vi "AIT 1553 Message Page.vi"(8 "error in (no error)":errorcluster, 11 "Node Ptr":T1 format="%.0x") -> (0 "error out":errorcluster)   [LabVIEW 2011, in "AIT 1553 Custom Device.lvlib"]
uses:
  AIT 1553 Custom Device.lvlib
  <vilib>/NI Veristand/Custom Device API/Custom Device Item Ref.ctl
  Controls and Global/Global.vi
  <vilib>/NI Veristand/Custom Device API/Get Item Property (U32 Array).vi
  <vilib>/NI Veristand/Custom Device API/Get Item Property (Boolean).vi
  <vilib>/NI Veristand/Custom Device API/Get Item Property (U16).vi
  <vilib>/NI Veristand/Custom Device API/Custom Device API.lvlib
panel:
  out "Default Message Buffer Data":u32[](array[numeric])
  out "Messge Buffer ID":u16
  out "RT Sub Address":u16
  out "RT Address":u16
  out "Message Type":string
  in  "Header":cluster{"Section Name":string}={"Section Name"="AIT 1553 Message"}
  in  "Description":string
  out "Name":string
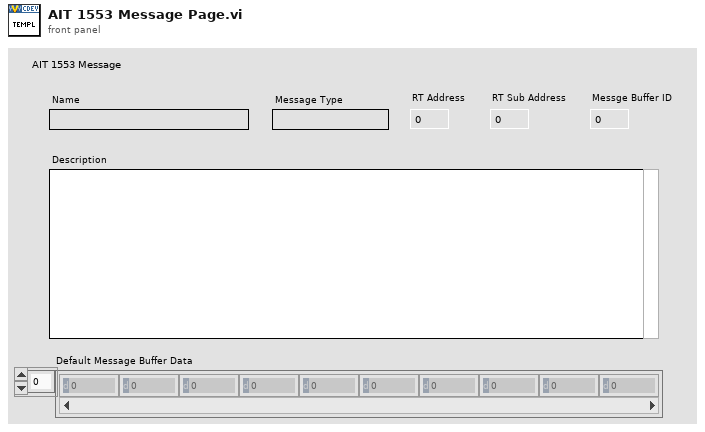
[diagram p1: front panel]
types:
  T1 = typedef "Custom Device API.lvlib/Custom Device Item Ref.ctl" = u64
  T2 = typedef "Custom Device API.lvlib/Custom Device Item Info.ctl" = cluster{"Name":string, "Is Channel":bool, "GUID":string}
  T3 = typedef "Custom Device API.lvlib/Custom Device Commands.ctl" = enum16{"Default", "Item renamed", "Shutdown", "Dynamic button pressed"}
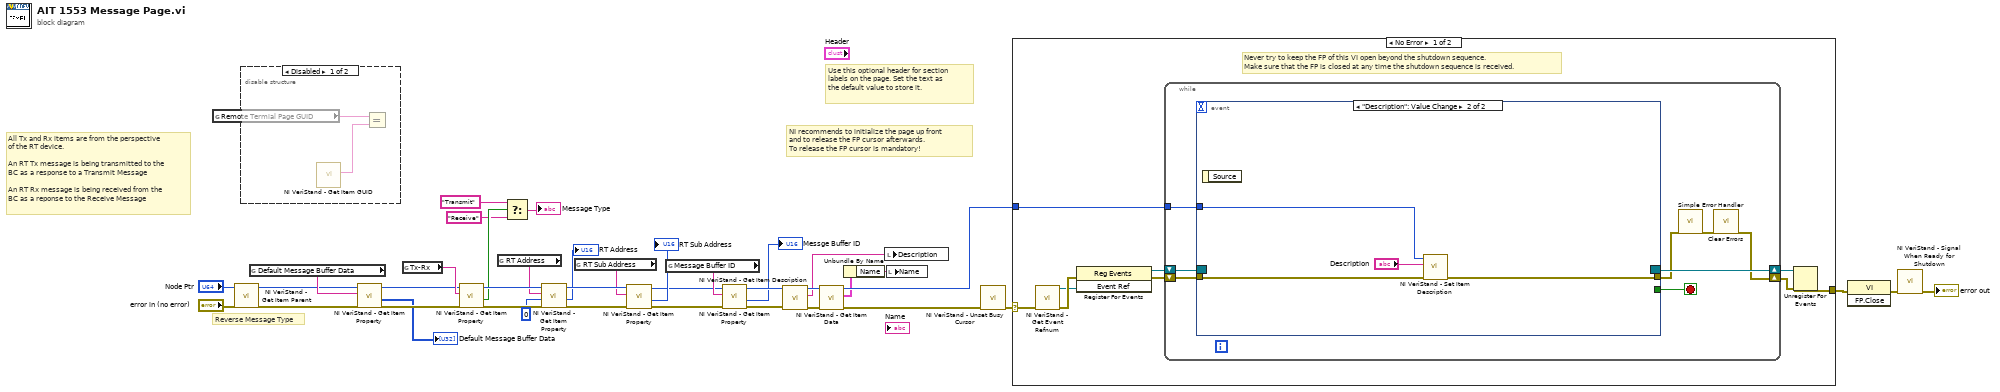
[diagram p0: block diagram]
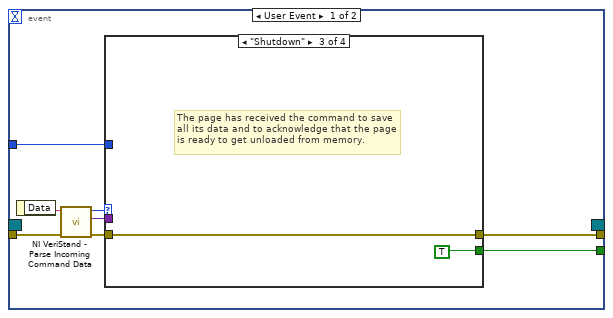
[diagram p3: hidden frame]
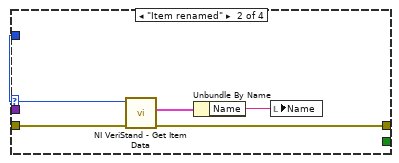
[diagram p5: hidden frame]
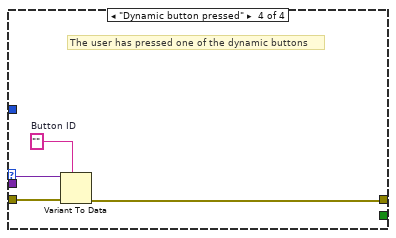
[diagram p6: hidden frame]
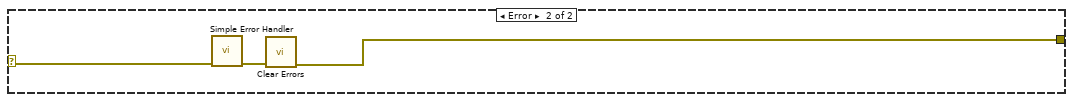
[diagram p7: hidden frame]
diagram:
  # "Reverse Message Type"
  # "All Tx and Rx items are from the perspective \nof the RT device.\n\nAn RT Tx message is being transmitted to the \nBC as a response to a Transmit Message\n\nAn RT Rx message is being received from the \nBC as a reponse to the Receive Message"
  # "Use this optional header for section labels on the page. Set the text as the default value to store it."
  # "NI recommends to initialize the page up front\nand to release the FP cursor afterwards.\nTo release the FP cursor is mandatory!"
  n1 = call <vilib>:"NI VeriStand - Get Item Parent.vi"("error in (no error)"="error in (no error)", "Item Ref in"="Node Ptr") -> ("error out"=w2:errorcluster, "Item Ref out"=w1:T1)  [unwired: 6 in, 2 out]
  n2 = disable-structure shown="Disabled" {
    frame Disabled {
      n3 = global read "Global.vi" "Remote Termial Page GUID"() -> (w40:string)
      n4 = call <vilib>:"NI VeriStand - Get Item GUID.vi"() -> ("GUID"=w41:string)  [unwired: 9 in, 2 out]
      n5 = Equal?(x=w40, y=w41) -> ()  [unwired: 1 out]
    }
    frame Enabled {
    }
  }
  n6 = global read "Global.vi" "Default Message Buffer Data"() -> (w5:string)
  n7 = call-poly <vilib>:"NI VeriStand - Get Item Property.vi"("error in (no error)"=w2, "Property Name"=w5, "Item Ref in"=w1) -> ("error out"=w6:errorcluster, "Value"=→"Default Message Buffer Data":u32[], "Item Ref out"=w4:T1)  [unwired: 5 in, 1 out]
  n8 = global read "Global.vi" "Tx-Rx"() -> (w7:string)
  n9 = call-poly <vilib>:"NI VeriStand - Get Item Property.vi"("error in (no error)"=w6, "Property Name"=w7, "Item Ref in"=w4) -> ("error out"=w27:errorcluster, "Value"=w22:bool, "Item Ref out"=w28:T1)  [unwired: 5 in, 1 out]
  n10 = global read "Global.vi" "RT Address"() -> (w18:string)
  n11 = Select(t="Transmit" ("Message Type"), s=w22, f="Receive" ("Message Type")) -> (s? t:f=→"Message Type":string)
  n12 = call-poly <vilib>:"NI VeriStand - Get Item Property.vi"("error in (no error)"=w27, "Default Value"=u16 0 ("RT Address"), "Property Name"=w18, "Item Ref in"=w28) -> ("error out"=w23:errorcluster, "Value"=→"RT Address":u16, "Item Ref out"=w24:T1)  [unwired: 4 in, 1 out]
  n13 = global read "Global.vi" "RT Sub Address"() -> (w14:string)
  n14 = call-poly <vilib>:"NI VeriStand - Get Item Property.vi"("error in (no error)"=w23, "Property Name"=w14, "Item Ref in"=w24) -> ("error out"=w13:errorcluster, "Value"=→"RT Sub Address":u16, "Item Ref out"=w9:T1)  [unwired: 5 in, 1 out]
  n15 = global read "Global.vi" "Message Buffer ID"() -> (w12:string)
  n16 = call-poly <vilib>:"NI VeriStand - Get Item Property.vi"("error in (no error)"=w13, "Property Name"=w12, "Item Ref in"=w9) -> ("error out"=w11:errorcluster, "Value"=→"Messge Buffer ID":u16, "Item Ref out"=w10:T1)  [unwired: 5 in, 1 out]
  n17 = call <vilib>:"NI VeriStand - Get Item Description.vi"("error in (no error)"=w11, "Item Ref in"=w10) -> ("error out"=w31:errorcluster, "Description"=w32:string, "Item Ref out"=w33:T1)  [unwired: 7 out]
  n18 = call <vilib>:"NI VeriStand - Get Item Data.vi"("error in (no error)"=w31, "Item Ref in"=w33) -> ("error out"=w36:errorcluster, "Item Info"=w30:T2, "Item Ref out"=w34:T1)  [unwired: 7 out]
  n19 = Unbundle By Name(w30) -> ("Name"=w29:string)
  n20 = local write "Description"(w32) -> ()
  n21 = local write "Name"(w29) -> ()
  n22 = call <vilib>:"NI VeriStand - Unset Busy Cursor.vi"("error in (no error)"=w36) -> ("error out"=w35:errorcluster)  [unwired: 10 out]
  n23 = case shown="No Error" w35 {
    selector: w35 -> [w42 w85]
    tunnel: [w47 w83] -> w39
    tunnel: w34 -> [w43 _]
    frame No Error {
      # "Never try to keep the FP of this VI open beyond the shutdown sequence.\nMake sure that the FP is closed at any time the shutdown sequence is received."
      n24 = call <vilib>:"NI VeriStand - Get Event Refnum.vi"("error in (no error)"=w42) -> ("error out"=w50:errorcluster, "Event Ref"=w46:refnum<user-event>)  [unwired: 9 out]
      n25 = register-events(error in=w50, w46) -> (reference out=w44:refnum<event-registration>, error out=w45:errorcluster)  [unwired: 1 in]
      n26 = while {
        tunnel: w43 -> [w54]
        shift-right: [w51] -> w48
        shift-left: w45 -> [w57]
        shift-right: [w58] -> w49
        shift-left: w44 -> [w56]
        stop <- w55 stop-if-true
        n27 = event shown="[1] \"Description\": Value Change" {
          selector: w56 -> [_ _]
          dyn-events: [_ _] -> w58
          timeout: _ -> [_ _]
          tunnel: w57 -> [w66 w81]
          tunnel: [w62 _] -> w55
          tunnel: [w61 w80] -> w53
          tunnel: w54 -> [w60 w82]
          event User Event {
            n28 = event-data() -> ("Data"=w65:string)  [unwired: 1 out]
            n29 = call <vilib>:"NI VeriStand - Parse Incoming Command Data.vi"("error in (no error)"=w66, "Incoming data"=w65) -> ("error out"=w64:errorcluster, "Outgoing data"=w59:variant, "Action"=w63:T3)  [unwired: 7 out]
            n30 = case shown="\"Shutdown\"" w63 {
              tunnel: w64 -> [w67 w72 w73 w78]
              tunnel: [_ _ TRUE _] -> w62
              tunnel: [w67 w69 w73 w75] -> w61
              tunnel: w60 -> [_ w71 _ _]
              tunnel: w59 -> [_ _ _ w77]
              frame "Default", Default {
              }
              frame "Item renamed" {
                n31 = call <vilib>:"NI VeriStand - Get Item Data.vi"("error in (no error)"=w72, "Item Ref in"=w71) -> ("error out"=w69:errorcluster, "Item Info"=w70:T2)  [unwired: 8 out]
                n32 = Unbundle By Name(w70) -> ("Name"=w68:string)
                n33 = local write "Name"(w68) -> ()
              }
              frame "Shutdown" {
                # "The page has received the command to save all its data and to acknowledge that the page is ready to get unloaded from memory."
              }
              frame "Dynamic button pressed" {
                w76 = ""  # Button ID
                # "The user has pressed one of the dynamic buttons"
                n34 = Variant To Data(error in=w78, type=w76, Variant=w77) -> (error out=w75:errorcluster)  [unwired: 1 out]
              }
            }
          }
          event "Description": Value Change {
            n35 = event-data() -> ()  [unwired: 2 out]
            n36 = call <vilib>:"NI VeriStand - Set Item Description.vi"("error in (no error)"=w81, "Description"="Description", "Item Ref in"=w82) -> ("error out"=w80:errorcluster)  [unwired: 8 out]
          }
        }
        n37 = call <vilib>:"Simple Error Handler.vi"("error in (no error)"=w53) -> ("error out"=w52:errorcluster)  [unwired: 1 in, 7 out]
        n38 = call <vilib>:"Clear Errors.vi"("error in (no error)"=w52) -> ("error out"=w51:errorcluster)  [unwired: 6 out]
      }
      n39 = Unregister For Events(event registration refnum=w49, error in=w48) -> (error out=w47:errorcluster)
    }
    frame Error {
      n40 = call <vilib>:"Simple Error Handler.vi"("error in (no error)"=w85) -> ("error out"=w84:errorcluster)  [unwired: 1 in, 7 out]
      n41 = call <vilib>:"Clear Errors.vi"("error in (no error)"=w84) -> ("error out"=w83:errorcluster)  [unwired: 6 out]
    }
  }
  n42 = invoke class="VI" method="FP.Close"(error in=w39) -> (error out=w38:errorcluster)  [unwired: 2 in, 2 out]
  n43 = call <vilib>:"NI VeriStand - Signal When Ready for Shutdown.vi"("error in (no error)"=w38) -> ("error out"=→"error out":errorcluster)  [unwired: 10 out]
